vi "Write Send Builder.vi"(10 "Message Maker.lvlib:Send Builder.lvclass":refnum<class "Send Builder.lvclass">, 11 "Message Scripter in":refnum<class "Message Scripter.lvclass">) -> (3 "Message Scripter out":refnum<class "Message Scripter.lvclass">)   [LabVIEW 2020, in "Message Maker.lvlib" / "Message Scripter.lvclass"]
uses:
  Message Scripter.lvclass
  Send Builder/Send Builder.lvclass
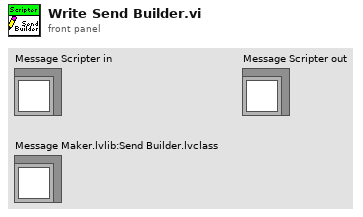
[diagram p1: front panel]
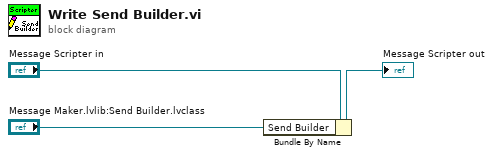
[diagram p0: block diagram]
diagram:
  n1 = Bundle By Name(cluster="Message Scripter in", "Send Builder"="Message Maker.lvlib:Send Builder.lvclass") -> (→"Message Scripter out":refnum<class "Message Scripter.lvclass">)
